vi "RTS Read Full Config File.vi"(8 "error in (no error)":errorcluster, 11 "Pattern":path) -> (0 "error out":errorcluster, 1 "Slide":T1[](array[typedef]) {"Start Time" format="%<%X\n%x>T"; "End Time" format="%<%X\n%x>T"}, 2 "Cab":T1[](array[typedef]) {"Start Time" format="%<%X\n%x>T"; "End Time" format="%<%X\n%x>T"}, 3 "Freezer":T1[](array[typedef]) {"Start Time" format="%<%X\n%x>T"; "End Time" format="%<%X\n%x>T"})   [LabVIEW 2016]
uses:
  Type Definitions/RTS Door Ops Client.ctl
  Type Definitions/RTS Door Opening Schedule.ctl
  Type Definitions/RTS Door Ops Sequence.ctl
  <vilib>/Utility/config.llb/NI_LVConfig.lvlib
panel:
  out "key names 3":string[][](array[string])
  out "key names 2":string[][](array[string])
  out "key names":string[][](array[string])
  # "Chamber Conditions:"
  # "Chamber Conditions:"
  # "Chamber Conditions:"
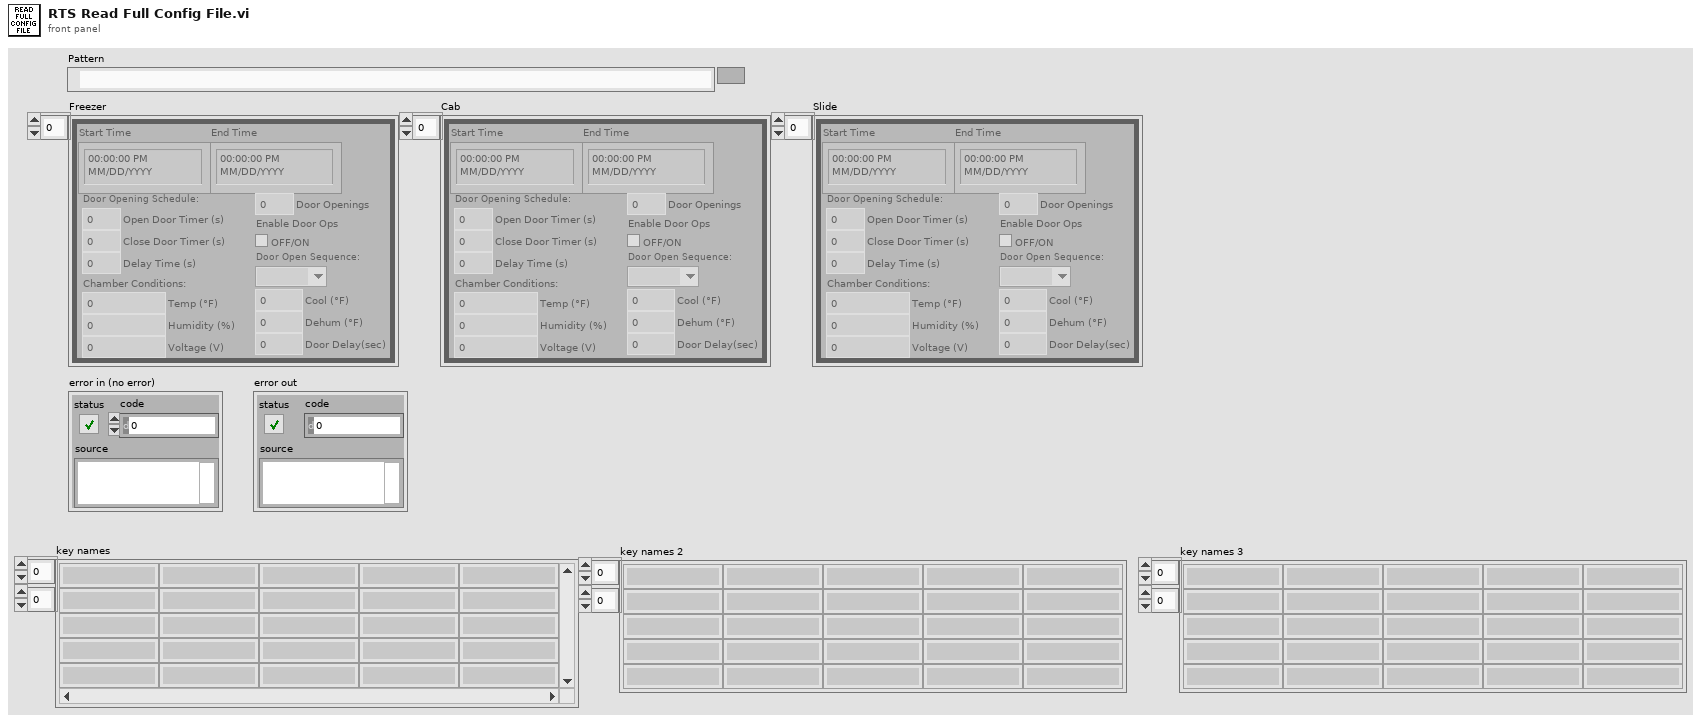
[diagram p1: front panel]
types:
  T1 = typedef "RTS Door Ops Client.ctl" = cluster{"End Time":timestamp, "Start Time":timestamp, "Door Opening Schedule:":T2, "Enable Door Ops":bool, "Door Openings":u32, "Temp (°F)":dbl, "Humidity (%)":dbl, "Voltage (V)":dbl, "Door Open Sequence:":T3, "Door Delay(sec)":dbl, "Dehum (°F)":dbl, "Cool (°F)":dbl}
  T2 = typedef "RTS Door Opening Schedule.ctl" = cluster{"Open Door Timer (s)":dbl, "Delay Time (s)":dbl, "Close Door Timer (s)":dbl}
  T3 = typedef "RTS Door Ops Sequence.ctl" = enum16{"", "1st", "2nd", "3rd"}
  T4 = typedef "NI_LVConfig.lvlib/Config Data RefNum.ctl" = refnum<k1>
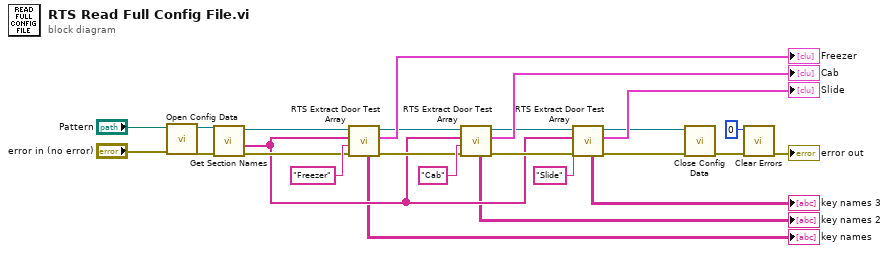
[diagram p0: block diagram]
diagram:
  n1 = call <vilib>:"Open Config Data.vi"("error in (no error)"="error in (no error)", "configuration file path"="Pattern") -> ("error out"=w10:errorcluster, "refnum"=w11:T4)  [unwired: 7 in, 1 out]
  n2 = call <vilib>:"Get Section Names.vi"("error in (no error)"=w10, "refnum"=w11) -> ("error out"=w13:errorcluster, "section names"=w9:string[], "refnum out"=w12:T4)  [unwired: 7 in]
  n3 = call "RTS Extract Door Test Array.vi"("error in (no error)"=w13, "Section Name"="Freezer" ("element"), "section names"=w9, "Refnum in"=w12) -> ("error out"=w17:errorcluster, "Array"=→"Freezer":T1[], "Refnum out"=w14:T4, "key names"=→"key names":string[][])  [unwired: 4 in]
  n4 = call "RTS Extract Door Test Array.vi"("error in (no error)"=w17, "Section Name"="Cab" ("element"), "section names"=w9, "Refnum in"=w14) -> ("error out"=w16:errorcluster, "Array"=→"Cab":T1[], "Refnum out"=w15:T4, "key names"=→"key names 2":string[][])  [unwired: 4 in]
  n5 = call "RTS Extract Door Test Array.vi"("error in (no error)"=w16, "Section Name"="Slide" ("element"), "section names"=w9, "Refnum in"=w15) -> ("error out"=w8:errorcluster, "Array"=→"Slide":T1[], "Refnum out"=w7:T4, "key names"=→"key names 3":string[][])  [unwired: 4 in]
  n6 = call <vilib>:"Close Config Data.vi"("error in (no error)"=w8, "refnum"=w7) -> ("error out"=w6:errorcluster)  [unwired: 8 in, 1 out]
  n7 = call <vilib>:"Clear Errors.vi"("error in (no error)"=w6, "specific error code to clear (0: all)"=0) -> ("error out"=→"error out":errorcluster)  [unwired: 4 in, 1 out]
